vi "TFC_Garage_LINESCAN.vi"() -> ()   [LabVIEW 2011]
uses:
  <vilib>/Platform/TimedLoop/XDataNode/timing_clust.ctl
  <vilib>/Platform/TimedLoop/XDataNode/nitl_modes.ctl
  <vilib>/Platform/TimedLoop/XDataNode/wakeup.ctl
  <vilib>/Instr/_visa.llb/VISA Configure Serial Port (Instr).vi
  <vilib>/Platform/TimedLoop/XDataNode/XDataNode.xnode
  <vilib>/Platform/TimedLoop/XDataNode/XDNodeRunTimeDep.lvlib
panel:
  in  "Hide Channel 1":bool
  in  "Hide Channel 0":bool
  in  "COM PORT":refnum<visa-resource-name>
  out "Output Command Queue":refnum<queue>
  out "Waveform Graph":dbl[][](graph)
  in  "?":bool
  out "Input Command Queue":refnum<queue>
  # "f"
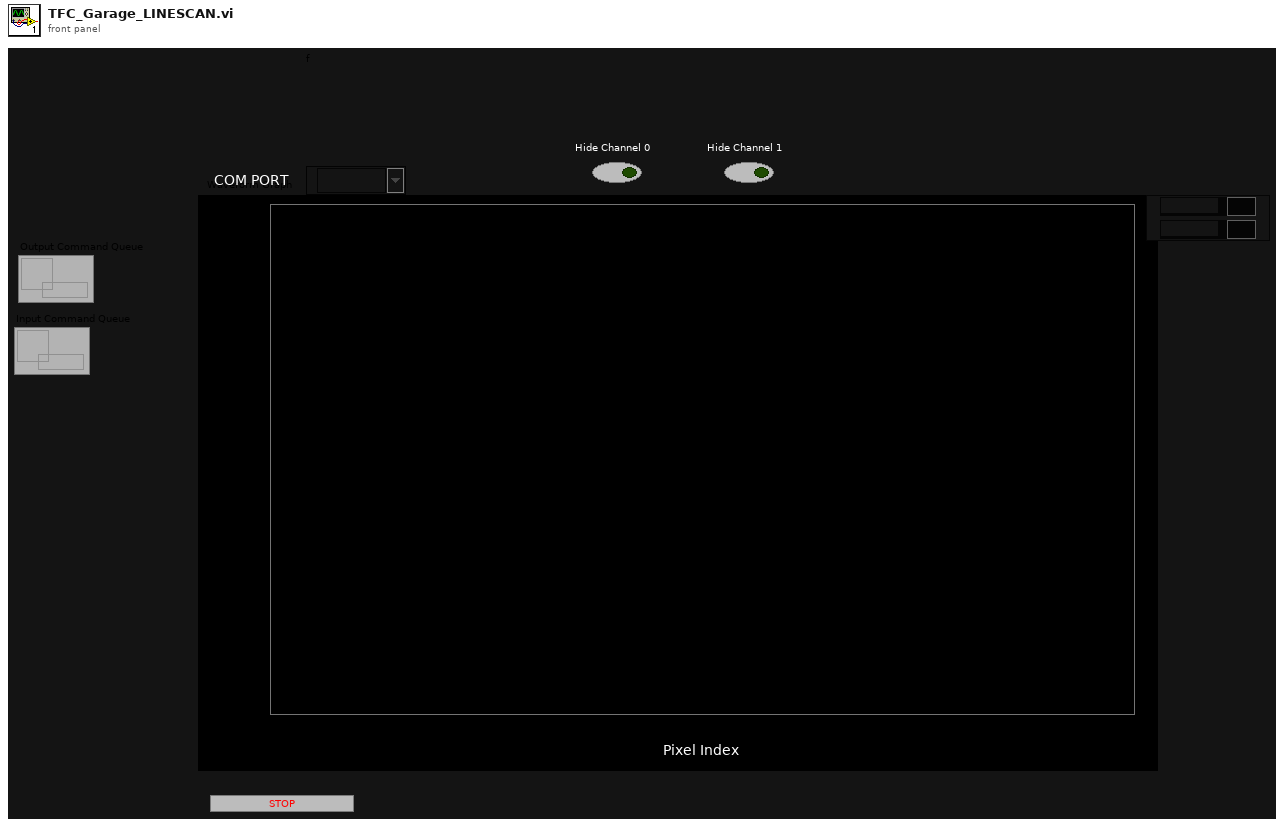
[diagram p1: front panel]
types:
  T1 = typedef "XDNodeRunTimeDep.lvlib/timing_clust.ctl" = cluster{"Expected End [f-1]":u64, "Actual End [f-1]":u64, "Finished Late? [f-1]":bool, "Expected End [i-1]":u64, "Actual End [i-1]":u64, "Finished Late? [i-1]":bool, "Expected Start [i]":u64, "Actual Start [i]":u64, "Expected Start [f]":u64, "Actual Start [f]":u64, "Source Name":string, "Structure Name":string, "Period":i64, "Deadline":i64, "Offset":i64, "Start":i64, "Priority":i32, "Timeout":i32, "Mode":T2, "Wakeup Reason":T3, "Error":errorcluster, "Source Type":string, "Secondary Source Type":string, "Global End Time":u64, "Global Start Time":u64, "Frame Duration":u64, "Iteration Duration":u64, "Assigned CPU":i32, "I/O Scan Engine Mode":u32}
  T2 = typedef "XDNodeRunTimeDep.lvlib/nitl_modes.ctl" = enum32{"No Change", "Process missed periods, maintain original phase", "Discard missed periods, maintain original phase", "Process missed periods, ignore original phase", "Discard missed periods, ignore original phase"}
  T3 = typedef "XDNodeRunTimeDep.lvlib/wakeup.ctl" = enum32{"Normal", "Aborted", "Asynchronous wakeup", "Timing source error", "Timed loop error", "Timeout"}
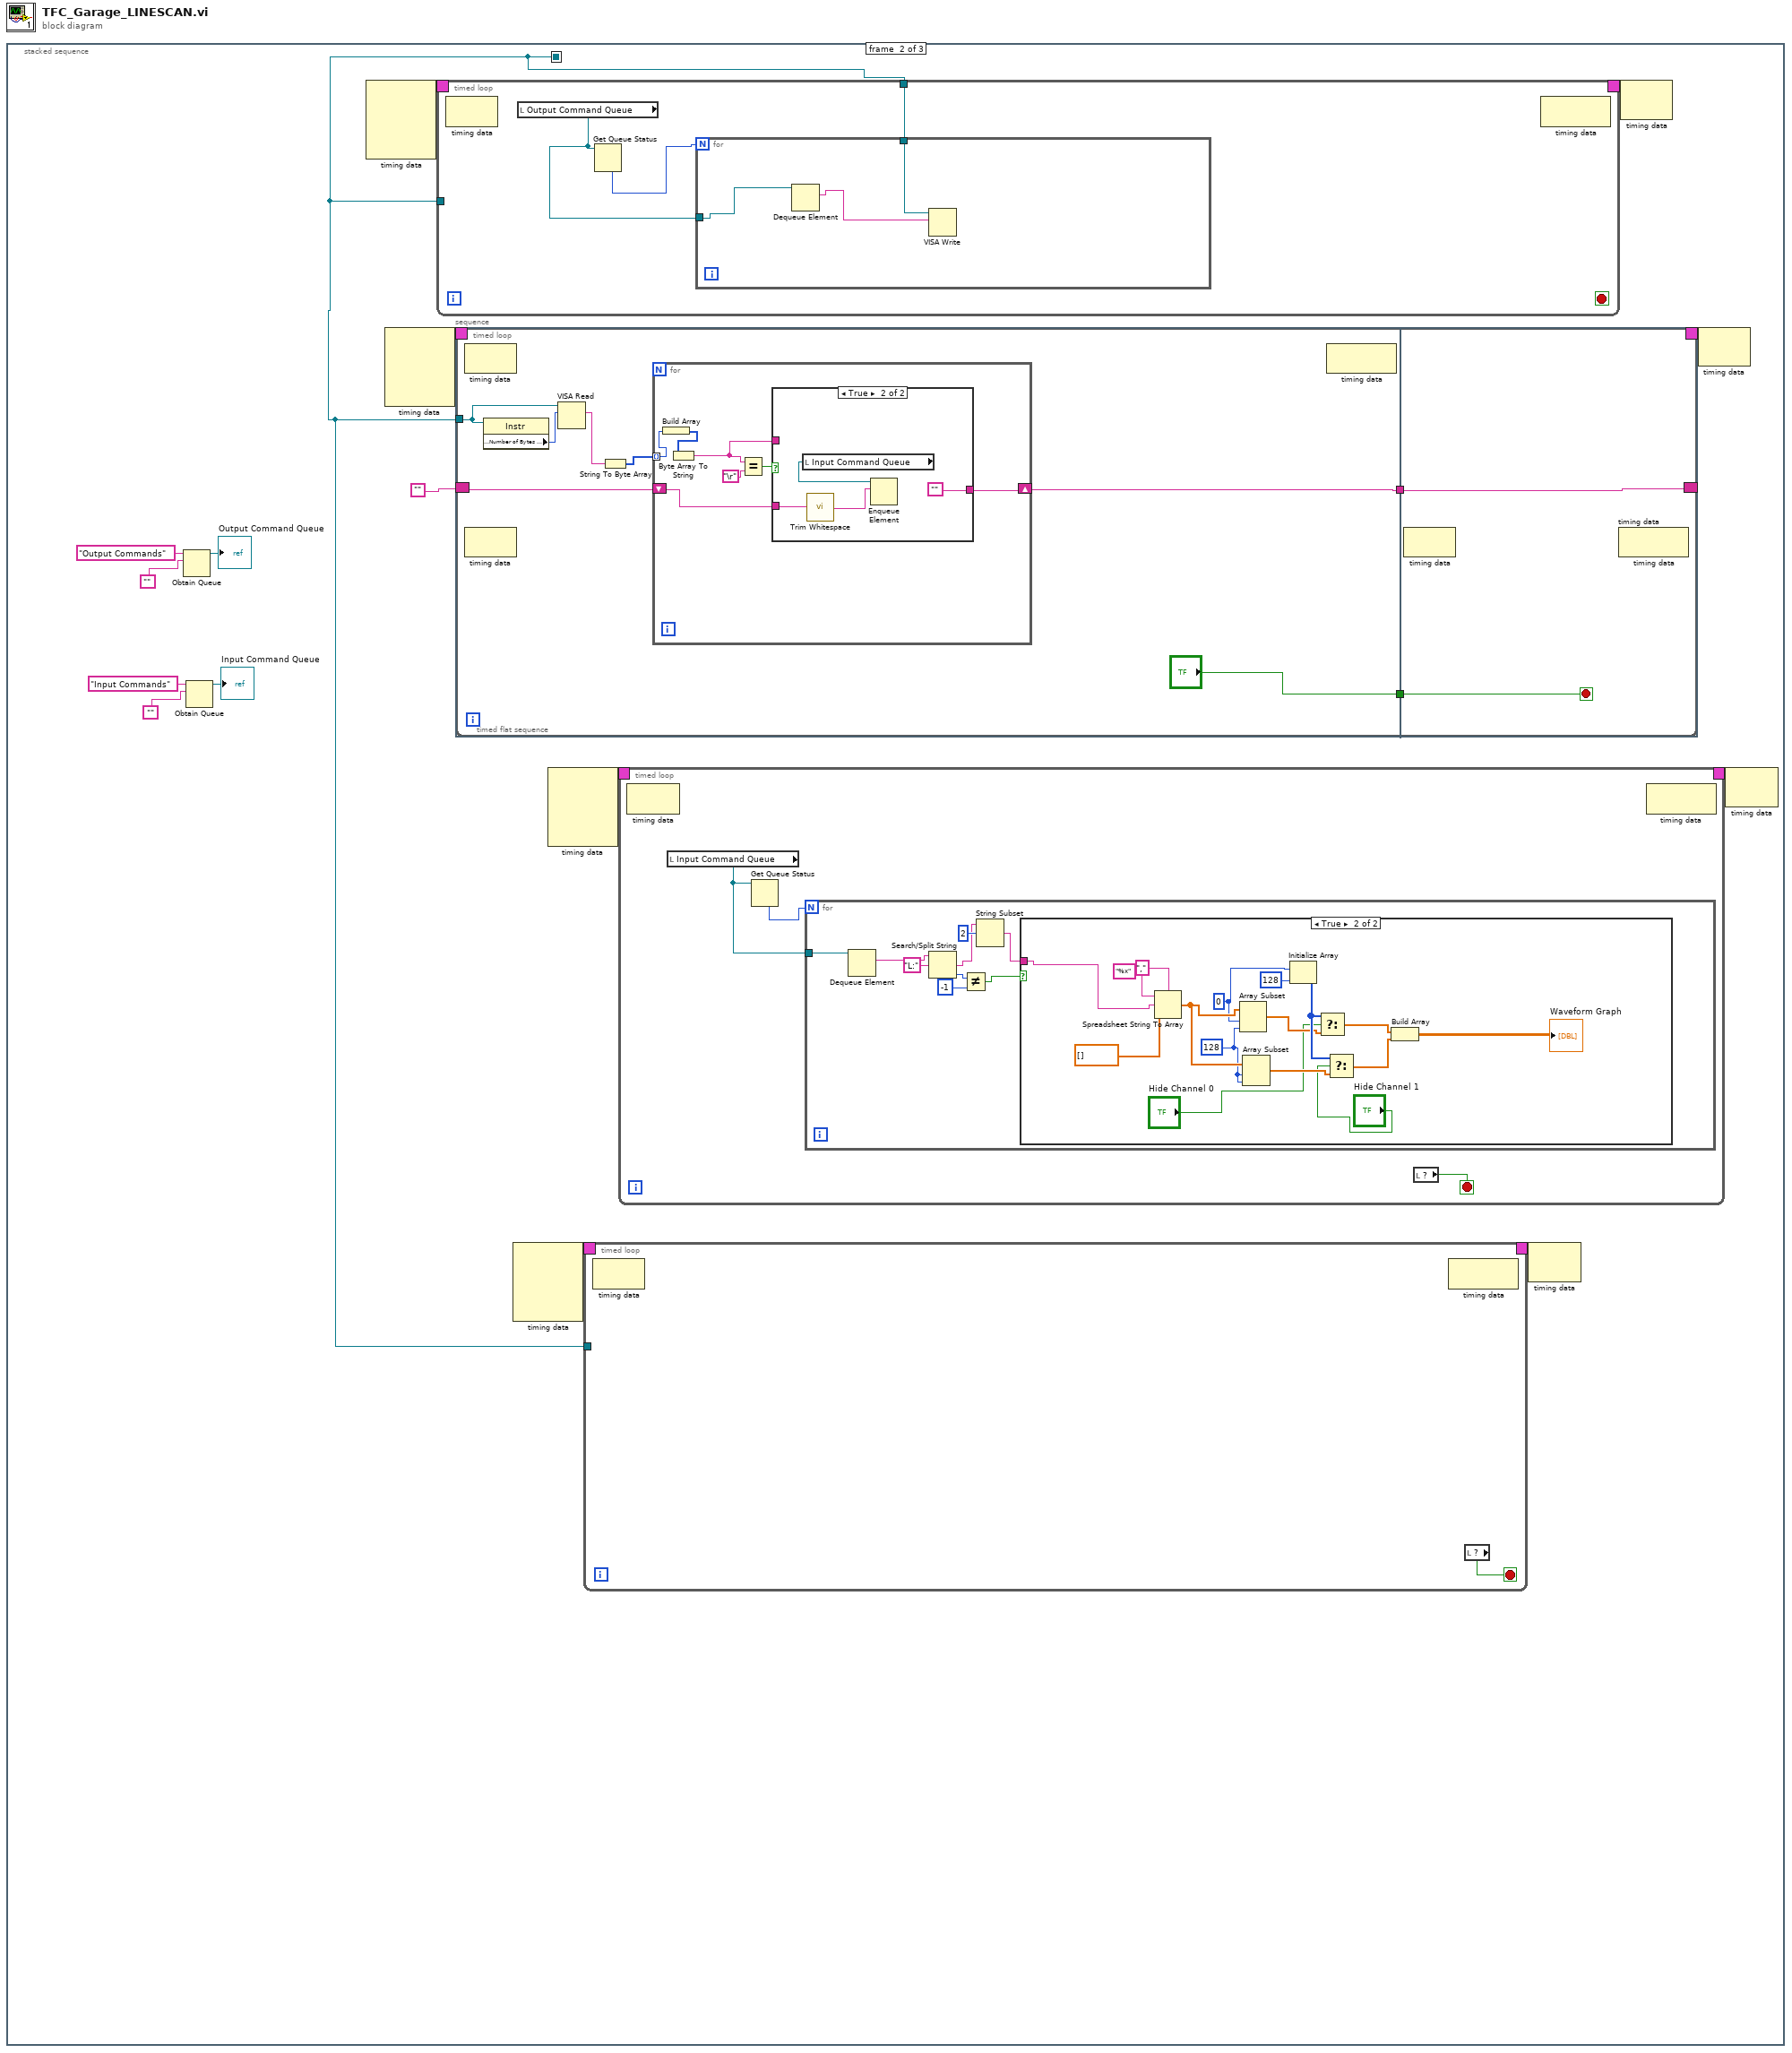
[diagram p0: block diagram]
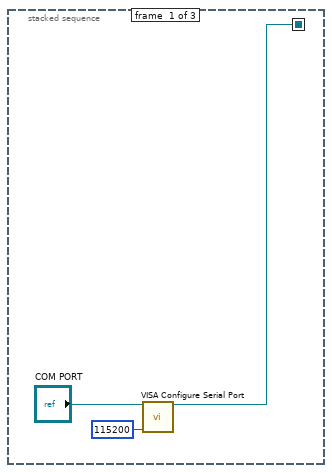
[diagram p2: hidden frame]
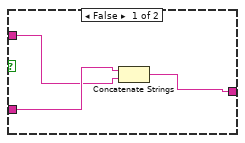
[diagram p4: hidden frame]
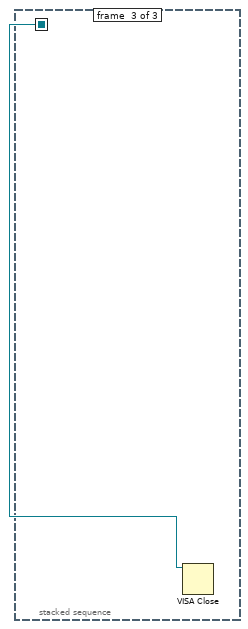
[diagram p5: hidden frame]
diagram:
  n1 = stacked-sequence {
    seq-local: [w3 _ _] -> [_ w4 w107]
    frame #0 {
      n2 = call-poly "VISA Configure Serial Port"("VISA resource name"="COM PORT", "baud rate (9600)"=u32 115200) -> ("VISA resource name out"=w3:refnum<visa-resource-name>)  [unwired: 12 in, 1 out]
    }
    frame #1 {
      n3 = Obtain Queue(name (unnamed)="Output Commands", element data type="") -> (queue out=→"Output Command Queue":refnum<queue>)  [unwired: 3 in, 2 out]
      n4 = Obtain Queue(name (unnamed)="Input Commands", element data type="") -> (queue out=→"Input Command Queue":refnum<queue>)  [unwired: 3 in, 2 out]
      n5 = node-c288() -> (w9:T1)  [unwired: 4 in]
      n6 = node-c288() -> (w19:T1)  [unwired: 4 in]
      n7 = timed-loop {
        timing: w9 -> [_]
        timing-out: [_] -> w8
        tunnel: w4 -> [w23]
        tunnel: [w23] -> _
        tunnel: w4 -> [w20]
        stop <- _ stop-if-true
        n8 = node-c288() -> ()  [unwired: 1 in, 1 out]
        n9 = local read "Output Command Queue"() -> (w21:refnum<queue>)
        n10 = Get Queue Status(queue=w21) -> (# elements in queue=w22:i32)  [unwired: 2 in, 7 out]
        n11 = for {
          N: w22 -> [_]
          tunnel: w21 -> [w26]
          tunnel: w20 -> [w25]
          n12 = Dequeue Element(queue=w26) -> (element=w24:string)  [unwired: 2 in, 3 out]
          n13 = VISA Write(VISA resource name=w25, write buffer=w24) -> ()  [unwired: 1 in, 3 out]
        }
        n14 = node-c288() -> ()  [unwired: 1 in, 1 out]
      }
      n15 = timed-loop {
        timing: w19 -> [_]
        timing-out: [_] -> w18
        shift-right: [w68] -> _
        shift-left: "" -> [w69]
        tunnel: w4 -> [w70]
        stop <- w99 stop-if-true
        n16 = timed-sequence {
          timing: _ -> [_]
          timing-out: _ -> [_]
          tunnel: w70 -> [w75]
          tunnel: w69 -> [w74]
          tunnel: [w73] -> w68
          n17 = timed-flat-sequence {
            tunnel: w75 -> [w78]
            tunnel: w74 -> [w82]
            tunnel: [w79] -> w72
            tunnel: ["?"] -> w71
            tunnel: [w100] -> w73
            tunnel: w72 -> [w100]
            tunnel: w71 -> [w99]
            frame #0 {
              n18 = node-c288() -> ()  [unwired: 1 in, 1 out]
              n19 = property class="Instr"(reference=w78) -> ("Serial Settings:Number of Bytes at Serial Port"=w77:u32)  [unwired: 1 in, 2 out]
              n20 = VISA Read(VISA resource name=w78, byte count=w77) -> (read buffer=w76:string)  [unwired: 1 in, 3 out]
              n21 = String To Byte Array(string=w76) -> (unsigned byte array=w80:u8[])
              n22 = for {
                tunnel: w80 -> [w84] mode=indexing
                shift-right: [w86] -> w79
                shift-left: w82 -> [w87]
                n23 = Build Array(w84) -> (w83:u8[])
                n24 = Byte Array To String(unsigned byte array=w83) -> (string=w85:string)
                n25 = Equal?(x=w85, y="\r") -> (x = y?=w88:bool)
                n26 = case shown="True" w88 {
                  tunnel: w87 -> [w92 w95]
                  tunnel: [w90 ""] -> w86
                  tunnel: w85 -> [w91 _]
                  frame False {
                    n27 = Concatenate Strings(w92, w91) -> (w90:string)
                  }
                  frame True {
                    n28 = local read "Input Command Queue"() -> (w96:refnum<queue>)
                    n29 = call <vilib>:"Trim Whitespace.vi"("string"=w95) -> ("trimmed string"=w94:string)  [unwired: 1 in]
                    n30 = Enqueue Element(queue=w96, element=w94) -> ()  [unwired: 2 in, 3 out]
                  }
                }
              }
              n31 = node-c288() -> ()  [unwired: 1 in, 1 out]
            }
            frame #1 {
              n32 = node-c288() -> ()  [unwired: 1 in, 1 out]
              n33 = node-c288() -> ()  [unwired: 1 in, 1 out]
            }
          }
        }
        n34 = node-c288() -> ()  [unwired: 1 in, 1 out]
        n35 = node-c288() -> ()  [unwired: 1 in, 1 out]
      }
      n36 = node-c288() -> (w15:T1)  [unwired: 4 in]
      n37 = node-c288() -> (w17:T1)  [unwired: 4 in]
      n38 = timed-loop {
        timing: w15 -> [_]
        timing-out: [_] -> w14
        tunnel: w4 -> [_]
        stop <- w31 stop-if-true
        n39 = node-c288() -> ()  [unwired: 1 in, 1 out]
        n40 = node-c288() -> ()  [unwired: 1 in, 1 out]
        n41 = local read item#1() -> (w31:bool)
      }
      n42 = timed-loop {
        timing: w17 -> [_]
        timing-out: [_] -> w16
        stop <- w36 stop-if-true
        n43 = node-c288() -> ()  [unwired: 1 in, 1 out]
        n44 = local read "Input Command Queue"() -> (w37:refnum<queue>)
        n45 = Get Queue Status(queue=w37) -> (# elements in queue=w38:i32)  [unwired: 2 in, 7 out]
        n46 = for {
          N: w38 -> [_]
          tunnel: w37 -> [w47]
          n47 = Dequeue Element(queue=w47) -> (element=w46:string)  [unwired: 2 in, 3 out]
          n48 = Search/Split String(string=w46, search string/char (-)="L:") -> (match + rest of string=w40:string, offset of match=w44:i32)  [unwired: 1 in, 1 out]
          n49 = Not Equal?(x=w44, y=-1) -> (x != y?=w42:bool)
          n50 = String Subset(string=w40, offset (0)=2) -> (substring=w39:string)  [unwired: 1 in]
          n51 = case shown="True" w42 {
            tunnel: w39 -> [_ w62]
            frame False {
            }
            frame True {
              w58 = 128 ("length")
              w55 = 0 ("index")
              n52 = Spreadsheet String To Array(delimiter (Tab)=",", format string="%x", spreadsheet string=w62, array type (2D Dbl)=dbl[] []) -> (array=w59:dbl[])
              n53 = Array Subset(array=w59, index=w55, length=w58) -> (w51:dbl[])
              n54 = Array Subset(array=w59, index=w58, length=w58) -> (w50:dbl[])
              n55 = Initialize Array(w55, 128 ("dimension size")) -> (w54:i32[])
              n56 = Select(t=w54, s="Hide Channel 0", f=w51) -> (s? t:f=w52:dbl[])
              n57 = Select(t=w54, s="Hide Channel 1", f=w50) -> (s? t:f=w53:dbl[])
              n58 = Build Array(w52, w53) -> (→"Waveform Graph":dbl[][])
            }
          }
        }
        n59 = local read item#1() -> (w36:bool)
        n60 = node-c288() -> ()  [unwired: 1 in, 1 out]
      }
      n61 = node-c288(w14) -> ()  [unwired: 1 out]
      n62 = node-c288(w8) -> ()  [unwired: 1 out]
      n63 = node-c288(w18) -> ()  [unwired: 1 out]
      n64 = node-c288(w16) -> ()  [unwired: 1 out]
    }
    frame #2 {
      n65 = VISA Close(VISA resource name=w107) -> ()  [unwired: 1 in, 1 out]
    }
  }
